vi "XY from 2D Commands.vi"(1 "Y 1D Array":dbl[](array[numeric])=[-10.0, -9.0, -8.0, -7.0, -6.0, -5.0, -4.0, -3.0, -2.0, -1.0, 0.0, 1.0, 2.0, 3.0, 4.0, 5.0, 6.0, 7.0, 8.0, 9.0, 10.0], 2 "2D wave":string="IV0_summ.itx.0000") -> (0 "wavenames":string[](array[string])=[" 'IV0_summ.itx.0000'[0][0]", " 'IV0_summ.itx.0000'[0][1]", " 'IV0_summ.itx.0000'[0][2]", " 'IV0_summ.itx.0000'[0][3]", " 'IV0_summ.itx.0000'[0][4]", " 'IV0_summ.itx.0000'[0][5]", " 'IV0_summ.itx.0000'[0][6]", " 'IV0_summ.itx.0000'[0][7]", " 'IV0_summ.itx.0000'[0][8]", " 'IV0_summ.itx.0000'[0][9]", " 'IV0_summ.itx.0000'[0][10]", " 'IV0_summ.itx.0000'[0][11]", " 'IV0_summ.itx.0000'[0][12]", " 'IV0_summ.itx.0000'[0][13]", " 'IV0_summ.itx.0000'[0][14]", " 'IV0_summ.itx.0000'[0][15]", " 'IV0_summ.itx.0000'[0][16]", " 'IV0_summ.itx.0000'[0][17]", " 'IV0_summ.itx.0000'[0][18]", " 'IV0_summ.itx.0000'[0][19]", " 'IV0_summ.itx.0000'[0][20]"])   [LabVIEW 2016, in "LV to ITX.lvclass"]
uses:
  LV to ITX.lvclass
panel:
  in  "input string 1":string="'#wave2D#'[][#i#]"
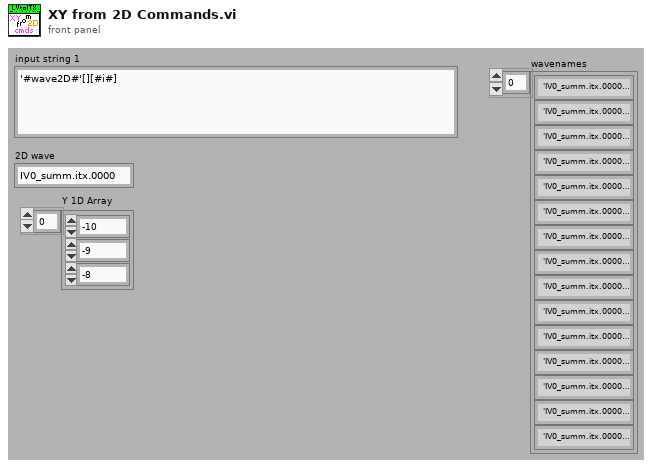
[diagram p1: front panel]
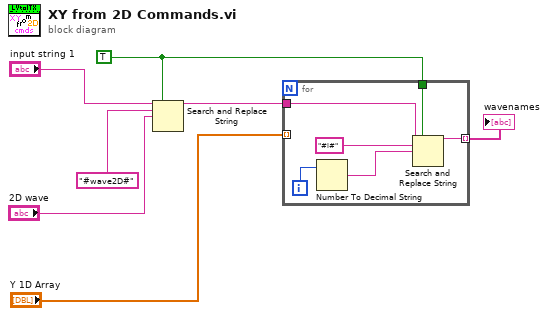
[diagram p0: block diagram]
diagram:
  w2 = TRUE ("replace all? (F)")
  n1 = Search and Replace String(replace all?=w2, input string="input string 1", search string="#wave2D#", replace string="2D wave") -> (result string=w3:string)  [unwired: 1 in, 6 out]
  n2 = for {
    tunnel: "Y 1D Array" -> [_] mode=indexing
    tunnel: w3 -> [w10]
    tunnel: w2 -> [w9]
    tunnel: [w8] -> w1 mode=indexing
    i -> [w13]
    n3 = Number To Decimal String(number=w13) -> (decimal integer string=w11:string)  [unwired: 1 out]
    n4 = Search and Replace String(replace all?=w9, input string=w10, search string="#i#", replace string=w11) -> (result string=w8:string)  [unwired: 1 in, 6 out]
  }
  "wavenames" <- w1
